vi "Read Controls of Panel from INI.vi"(8 "error in (no error)":errorcluster, 10 "VI Ref (calling VI)":refnum<vi>, 11 "refnum":T1) -> (0 "error out":errorcluster, 3 "refnum out":T1)   [LabVIEW 2017]
doc: "Reads the values of the front panel controls of VI Ref from a standard LabVIEW configuration (INI) file. Use it together with Write Controls of Panel to INI.vi."
uses:
  <vilib>/Utility/config.llb/Config Data RefNum.ctl
  _OpenG Variant Configuration File/OpenG Variant Configuration File.lvlib
  <vilib>/Utility/config.llb/NI_LVConfig.lvlib
panel:
  # "Read Panel from INI.vi\n\nReads all Front Panel data from INI file.\n\nPlease visit http://www.OpenG.org to learn about the\nOpen Source LabVIEW software movement.\n\nNOTICE -- YOU MUST LEAVE THIS NOTICE IN PLACE.  PER THE TERMS OF THE LICENSE BELOW, YOU MAY SUBLICENSE THIS SOFTWARE \nIN ANY WAY THAT DOES NOT CONFLICT WITH THIS LICENSE.\n\n### BSD License (http://www.opensource.org/licenses/bsd-license.php) Begin ###\n \nCopyright (c) 2002, Jean-Pierre Drolet <drolet_jp@hotmail.com>\n\nAll rights reserved.\n\nRedistribution and use in source and binary forms, with or without modification, are permitted provided that the following conditions are met:\n\n    * Redistributions of source code must retain the above copyright notice, this list of conditions and the following disclaimer.\n    * Redistributions in binary form must reproduce the above copyright notice, this list of conditions and the following disclaimer in the \n       documentation and/or other materials provided with the distribution.\n    * Neither the name of SciWare, James Kring, Inc., nor the names of its contributors may be used to endorse or promote products derived \n       from this software without specific prior written permission.\n\nTHIS SOFTWARE IS PROVIDED BY THE COPYRIGHT HOLDERS AND CONTRIBUTORS \"AS IS\" AND ANY EXPRESS OR IMPLIED WARRANTIES, \nINCLUDING, BUT NOT LIMITED TO, THE IMPLIED WARRANTIES OF MERCHANTABILITY AND FITNESS FOR A PARTICULAR PURPOSE ARE \nDISCLAIMED. IN NO EVENT SHALL THE COPYRIGHT OWNER OR CONTRIBUTORS BE LIABLE FOR ANY DIRECT, INDIRECT, INCIDENTAL,\n SPECIAL, EXEMPLARY, OR CONSEQUENTIAL DAMAGES (INCLUDING, BUT NOT LIMITED TO, PROCUREMENT OF SUBSTITUTE GOODS OR \nSERVICES; LOSS OF USE, DATA, OR PROFITS; OR BUSINESS INTERRUPTION) HOWEVER CAUSED AND ON ANY THEORY OF LIABILITY, \nWHETHER IN CONTRACT, STRICT LIABILITY, OR TORT (INCLUDING NEGLIGENCE OR OTHERWISE) ARISING IN ANY WAY OUT OF THE USE \nOF THIS SOFTWARE, EVEN IF ADVISED OF THE POSSIBILITY OF SUCH DAMAGE.\n\n### BSD License End ###"
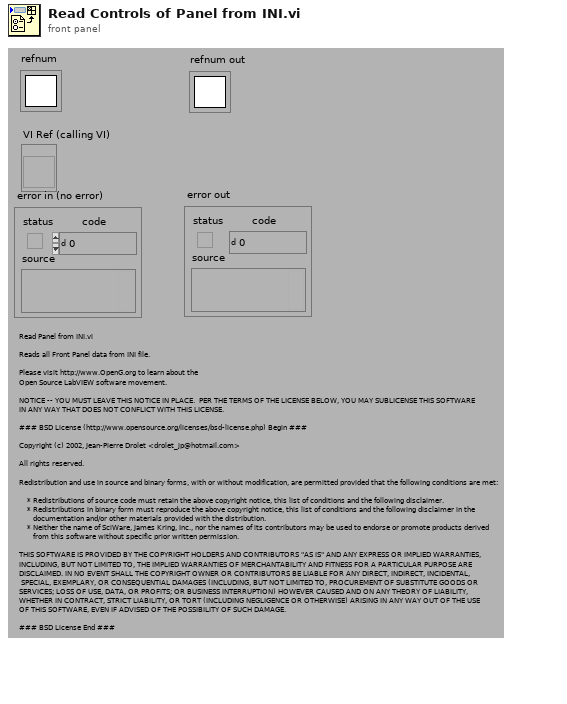
[diagram p1: front panel]
types:
  T1 = typedef "NI_LVConfig.lvlib/Config Data RefNum.ctl" = refnum<k1>
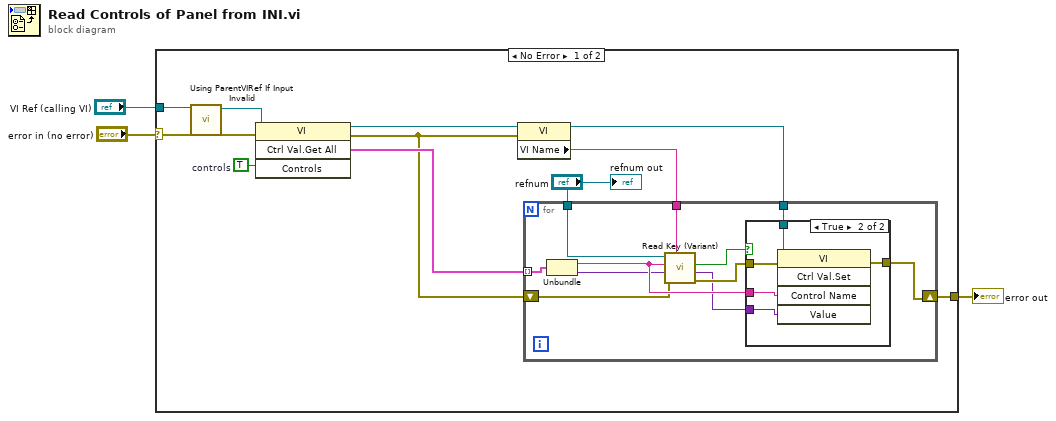
[diagram p0: block diagram]
diagram:
  n1 = case shown="No Error" "error in (no error)" {
    selector: "error in (no error)" -> [w8 w32]
    tunnel: [w7 w32] -> w2
    tunnel: "VI Ref (calling VI)" -> [w5 _]
    frame No Error {
      w14 = TRUE  # controls
      n2 = call "Using ParentVIRef If Input Invalid.vi"("VI Ref (calling VI)"=w5) -> ("VI Ref"=w4:refnum<vi>)  [unwired: 5 in, 1 out]
      n3 = invoke on="Invoke Node" class="VI" method="Ctrl Val.Get All"(reference=w4, error in=w8, "Controls"=w14) -> (reference out=w13:refnum<vi>, error out=w11:errorcluster, "Get All Control Values Variant"=w12:cluster{"Name":string, "Variant Data":variant}[])  [unwired: 1 in, 1 out]
      n4 = property on="Property Node" class="VI"(reference=w13, error in=w11) -> (reference out=w6:refnum<vi>, "VI Name"=w10:string)  [unwired: 1 out]
      n5 = for {
        tunnel: w12 -> [w25] mode=indexing
        tunnel: w10 -> [w24]
        tunnel: "refnum" -> [w23]
        shift-right: [w21] -> w7
        shift-left: w11 -> [w17]
        tunnel: w6 -> [w22]
        n6 = Unbundle(w25) -> ("Name"=w19:string, "Variant Data"=w18:variant)
        n7 = call "Read Key (Variant).vi"("section"=w24, "error in (no error)"=w17, "type"=w18, "key (optional)"=w19, "refnum"=w23) -> ("error out"=w20:errorcluster, "key-value"=w16:variant, "found?"=w15:bool)  [unwired: 3 in, 1 out]
        n8 = case shown="True" w15 {
          tunnel: w22 -> [_ w31]
          tunnel: [w26 w30] -> w21
          tunnel: w20 -> [w26 w29]
          tunnel: w19 -> [_ w28]
          tunnel: w16 -> [_ w27]
          frame False {
          }
          frame True {
            n9 = invoke class="VI" method="Ctrl Val.Set"(reference=w31, error in=w29, "Control Name"=w28, "Value"=w27) -> (error out=w30:errorcluster)  [unwired: 1 in, 4 out]
          }
        }
      }
      "refnum out" <- "refnum"
    }
    frame Error {
    }
  }
  "error out" <- w2
